vi "Write String Assertion.vi"(8 "error in (no error)":errorcluster, 10 "String Assertion":T1, 11 "String Assertion in":refnum<class "String Assertion.lvclass">) -> (0 "error out":errorcluster, 3 "String Assertion out":refnum<class "String Assertion.lvclass">)   [LabVIEW 2020, in "MacroAssert.lvlib" / "String Assertion.lvclass"]
uses:
  String Assertion.lvclass
  String Assertion.lvclass/String Assertion.ctl
  String Assertion Type.ctl
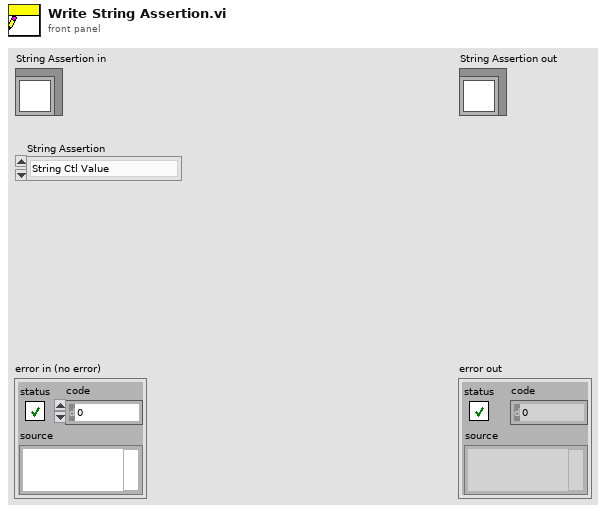
[diagram p1: front panel]
types:
  T1 = typedef "MacroAssert.lvlib/String Assertion.lvclass/String Assertion Type.ctl" = enum16{"String Ctl Value", "Ctl Caption Property", "Ctl Tip Strip Property", "Frontmost Window Name", "Frontmost VI Name"}
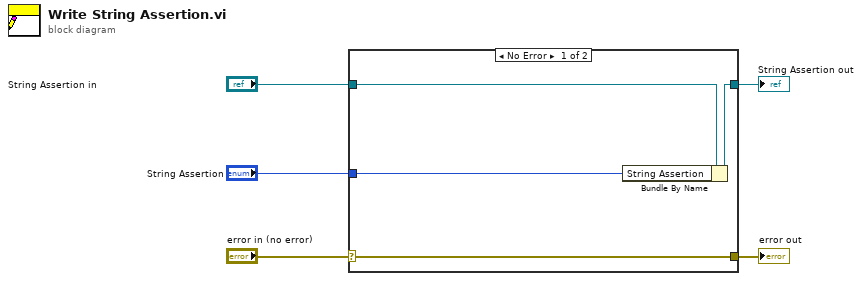
[diagram p0: block diagram]
diagram:
  n1 = case shown="No Error" "error in (no error)" {
    selector: "error in (no error)" -> [w9 w10]
    tunnel: [w9 w10] -> w4
    tunnel: [w7 w11] -> w2
    tunnel: "String Assertion in" -> [w8 w11]
    tunnel: "String Assertion" -> [w6 _]
    frame No Error {
      n2 = Bundle By Name(cluster=w8, "String Assertion"=w6) -> (w7:refnum<class "String Assertion.lvclass">)
    }
    frame Error {
    }
  }
  "error out" <- w4
  "String Assertion out" <- w2
